vi "Data_base_client.vi"(4 "Average Sampling freq":sgl=100.0 format="%.1f", 5 "Channels from Client":string[][](array[string])=[["Data Base:Measurement:Type", "LDA & Cw"], ["Data Base:Position:No of Inst", "2"], ["Data Base:Position:X1", "-60"], ["Data Base:Position:X2", ""], ["Data Base:Position:Y1", "2"], ["Data Base:Position:Y2", "0.00"], ["Data Base:Position:Z1", "0.00"], ["Data Base:Position:Z2", "2.00"]], 6 "Average Meas Time (min)":dbl=100.0 format="%.1f", 7 "End time":dbl, 8 "Start time":dbl, 9 "Results File Pathname":path, 10 "Raw Data Pathname":path) -> (1 "spreadsheet string":string, 2 "Channel values":string[](array[string]), 3 "Channel names":string[](array[string]))   [LabVIEW 2010]
doc: "This is an example of using features of the VI Server as a client. It shows how you might browse from one or more applications that may be exporting data from one or more data stations. \n\nThe example shows how to query a server for its list of exported VIs, how to get references to the VIs, and how call them with the Call By Reference function."
uses:
  Anemometry/Anemometry Sub Vis/Globals/Preference_global.vi
panel:
  out "Iterations":i32
  in  "Data Base server type":refnum<vi>
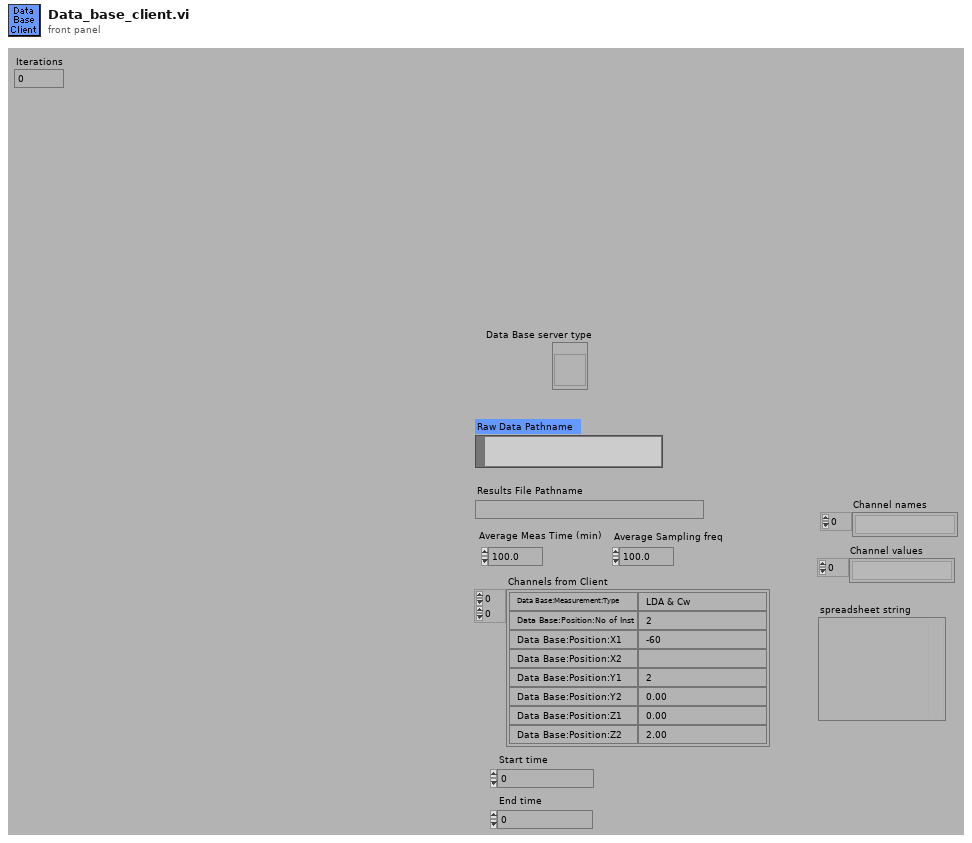
[diagram p1: front panel]
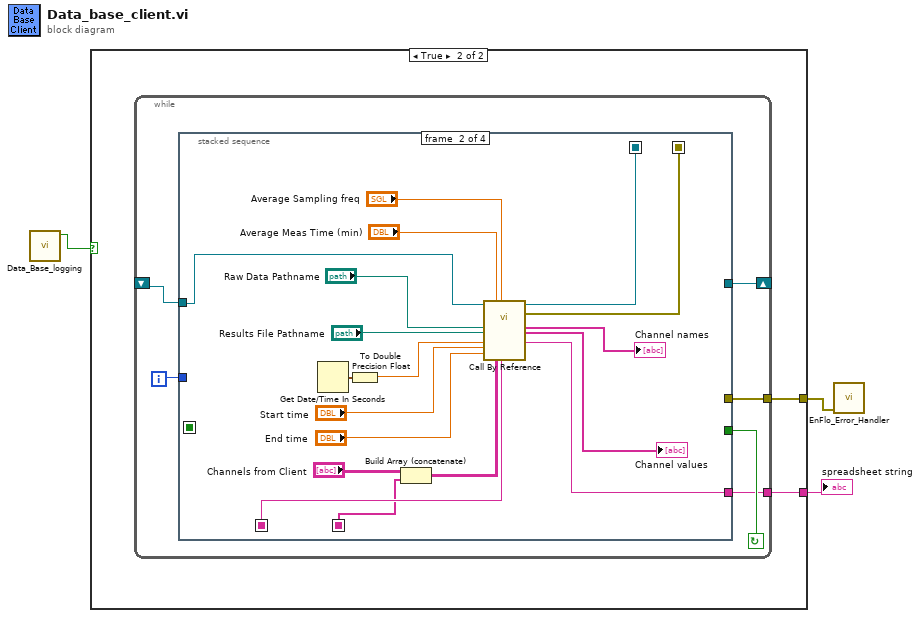
[diagram p0: block diagram]
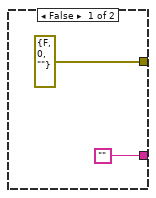
[diagram p2: hidden frame]
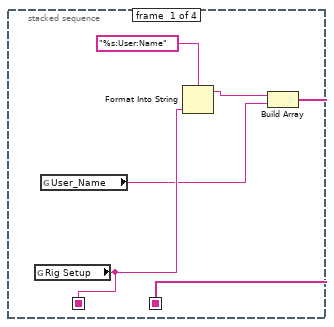
[diagram p3: hidden frame]
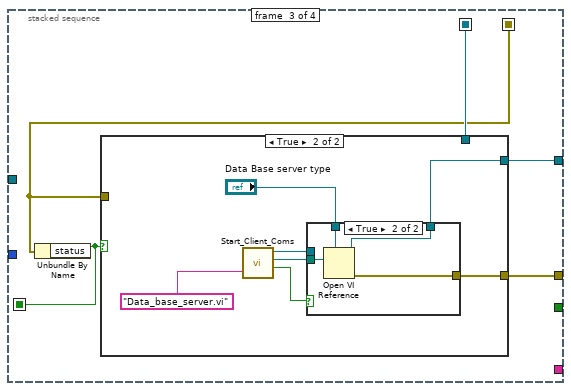
[diagram p4: hidden frame]
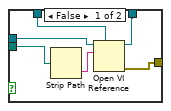
[diagram p6: hidden frame]
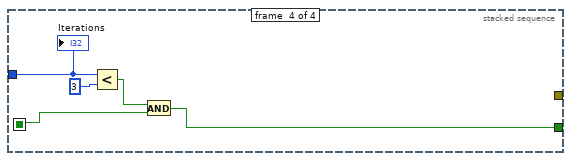
[diagram p7: hidden frame]
diagram:
  n1 = call "Data_Base_logging.vi"() -> ("Logging On?"=w1:bool)  [unwired: 4 out]
  n2 = case shown="True" w1 {
    tunnel: [errorcluster {"status"=FALSE, "code"=0, "source"=""} w7] -> w3
    tunnel: ["" w6] -> w2
    frame False {
    }
    frame True {
      n3 = while {
        tunnel: [w8] -> w6
        tunnel: [w9] -> w7
        shift-left: _ -> [w13]
        shift-right: [w12] -> _
        i -> [w11]
        stop <- w10 continue-if-true
        n4 = stacked-sequence {
          seq-local: [_ w29 _ _] -> [_ _ w40 _]
          seq-local: [_ w28 _ _] -> [_ _ w37 _]
          seq-local: [_ _ w39 _] -> [_ _ _ w62]
          seq-local: [w18 _ _ _] -> [_ w22 _ _]
          seq-local: [w14 _ _ _] -> [_ w19 _ _]
          tunnel: w13 -> [_ w30 _ _]
          tunnel: [_ _ w41 _] -> w12
          tunnel: w11 -> [_ _ _ w63]
          tunnel: [_ _ _ w61] -> w10
          tunnel: [_ _ w38 _] -> w9
          tunnel: [_ w25 _ _] -> w8
          frame #0 {
            n5 = global read "Preference_global.vi" "Rig Setup"() -> (w18:string)
            n6 = global read "Preference_global.vi" "User_Name"() -> (w15:string)
            n7 = Format Into String(format string="%s:User:Name", w18) -> (resulting string=w16:string)  [unwired: 2 in, 1 out]
            n8 = Build Array(w16, w15) -> (w14:string[])
          }
          frame #1 {
            n9 = Get Date/Time In Seconds() -> (seconds since 1Jan1904=w23:timestamp)
            n10 = To Double Precision Float(number=w23) -> (double precision float=w32:dbl)
            n11 = Build Array (concatenate)("Channels from Client", w19) -> (w20:string[][])
            n12 = call-by-ref "?"(reference=w30, "Results file"="Raw Data Pathname", "Data Base Pathname"="Results File Pathname", "Clients time"=w32, "Start time"="Start time", "End time"="End time", "Average Meas Time (min)"="Average Meas Time (min)", "Channels from Client"=w20, "Average Sampling freq"="Average Sampling freq", "Rig Name"=w22) -> (reference out=w29:refnum<vi>, error out=w28:errorcluster, "Channel names"=→"Channel names":string[], "Channel values"=→"Channel values":string[], "spreadsheet string"=w25:string)  [unwired: 9 in]
          }
          frame #2 {
            n13 = Unbundle By Name(w37) -> ("status"=w39:bool)
            n14 = case shown="True" w39 {
              tunnel: [w43 w46] -> w41
              tunnel: w40 -> [w43 _]
              tunnel: [w42 w44] -> w38
              tunnel: w37 -> [w42 _]
              frame False {
              }
              frame True {
                n15 = call "Start_Client_Coms.vi"("VI name to run on server"="Data_base_server.vi") -> ("LabVIEW application reference"=w48:refnum<vi>, "Checked VI name"=w49:path, "Local Call"=w47:bool)  [unwired: 1 in, 1 out]
                n16 = case shown="True" w47 {
                  tunnel: [w52 w60] -> w46
                  tunnel: "Data Base server type" -> [w53 w59]
                  tunnel: w49 -> [w55 w58]
                  tunnel: w48 -> [w54 _]
                  tunnel: [w51 w57] -> w44
                  frame False {
                    n17 = Strip Path(path=w55) -> (name=w56:string)  [unwired: 1 out]
                    n18 = Open VI Reference(type specifier VI Refnum (for type only)=w53, application reference (local)=w54, vi path=w56) -> (vi reference=w52:refnum<vi>, error out=w51:errorcluster)  [unwired: 1 in, 2 out]
                  }
                  frame True {
                    n19 = Open VI Reference(type specifier VI Refnum (for type only)=w59, vi path=w58) -> (vi reference=w60:refnum<vi>, error out=w57:errorcluster)  [unwired: 1 in, 3 out]
                  }
                }
              }
            }
          }
          frame #3 {
            n20 = Less?(x=w63, y=3) -> (x < y?=w65:bool)
            n21 = And(x=w65, y=w62) -> (x .and. y?=w61:bool)
            "Iterations" <- w63
          }
        }
      }
    }
  }
  "spreadsheet string" <- w2
  n22 = call "EnFlo_Error_Handler.vi"("error in (no error)"=w3) -> ()  [unwired: 2 in, 3 out]
